vi "Command to Analog Output.vi"() -> ()   [LabVIEW 2019, in "Part of Main VIs.lvlib" / "Command Library.lvlib"]
uses:
  <vilib>/DAQmx/write.llb/DAQmx Write (Analog DBL 1Chan 1Samp).vi
  <extravilib>/ChannelInstances/Tag-bool/Write With Abort.vi
  <extravilib>/ChannelInstances/Tag-str/Write With Abort.vi
  <extravilib>/ChannelInstances/Tag-bool/Read With Abort.vi
  <extravilib>/ChannelInstances/Tag-str/Read With Abort.vi
  <extravilib>/ChannelInstances/Tag-dbl/Write With Abort.vi
  <extravilib>/ChannelInstances/Tag-dbl/Read With Abort.vi
  <extravilib>/ChannelInstances/Tag-str/Instantiate.vi
  <extravilib>/ChannelInstances/Tag-dbl/Instantiate.vi
  <extravilib>/ChannelInstances/Tag-bool/Instantiate.vi
  <extravilib>/ChannelInstances/Tag-bool/EndpointRead.vi
  <extravilib>/ChannelInstances/Tag-str/EndpointRead.vi
  <extravilib>/ChannelInstances/Tag-dbl/Endpoint.vi
  <extravilib>/ChannelInstances/Tag-str/Endpoint.vi
  <vilib>/DAQmx/create/channels.llb/DAQmx Create Channel (AO-Voltage-Basic).vi
  <extravilib>/ChannelInstances/Tag-dbl/EndpointRead.vi
  <vilib>/DAQmx/miscellaneous.llb/DAQmx Fill In Error Info.vi
  <extravilib>/ChannelInstances/Tag-bool/Endpoint.vi
  Command Library.lvlib
  <extravilib>/ChannelInstances/Tag-bool.lvlib
  <resource>/objmgr/daqmx.rc
  <extravilib>/ChannelInstances/Tag-dbl.lvlib
  <extravilib>/ChannelInstances/Tag-str.lvlib
panel:
  out "Numeric 2":dbl
  in  "Numeric":dbl
  out "Waveform Chart":waveform(dbl)(graph)
  in  "stop":bool
  in  "String":string
  out "InterfaceName":string
  out "Voltage Value":dbl format="%e"
  out "BoardName":string
  out "ChannelNo":string
  out "Status":string
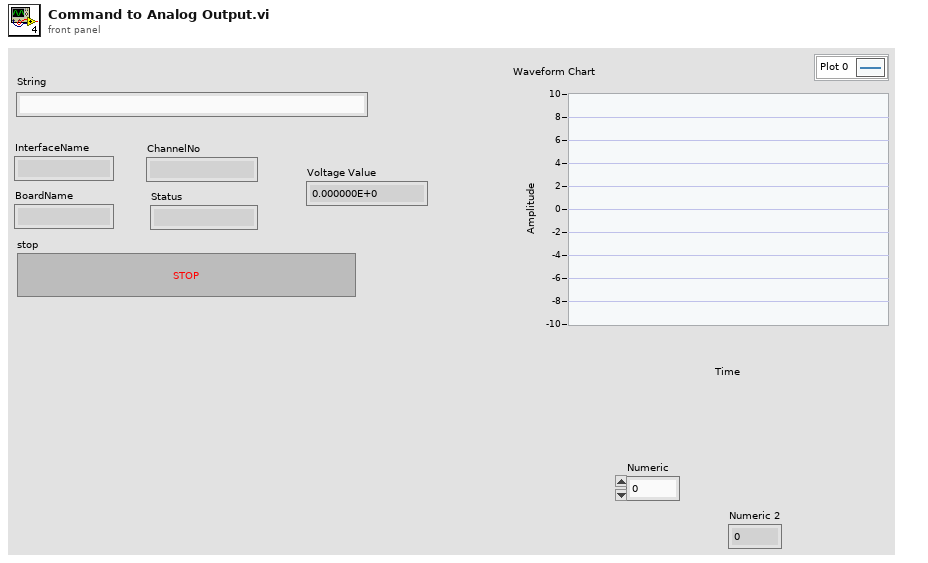
[diagram p1: front panel]
types:
  T1 = typedef "Tag-str.lvlib/))Channel.ctl" = refnum<queue>
  T2 = typedef "Tag-bool.lvlib/))Channel.ctl" = refnum<queue>
  T3 = typedef "Tag-dbl.lvlib/))Channel.ctl" = refnum<queue>
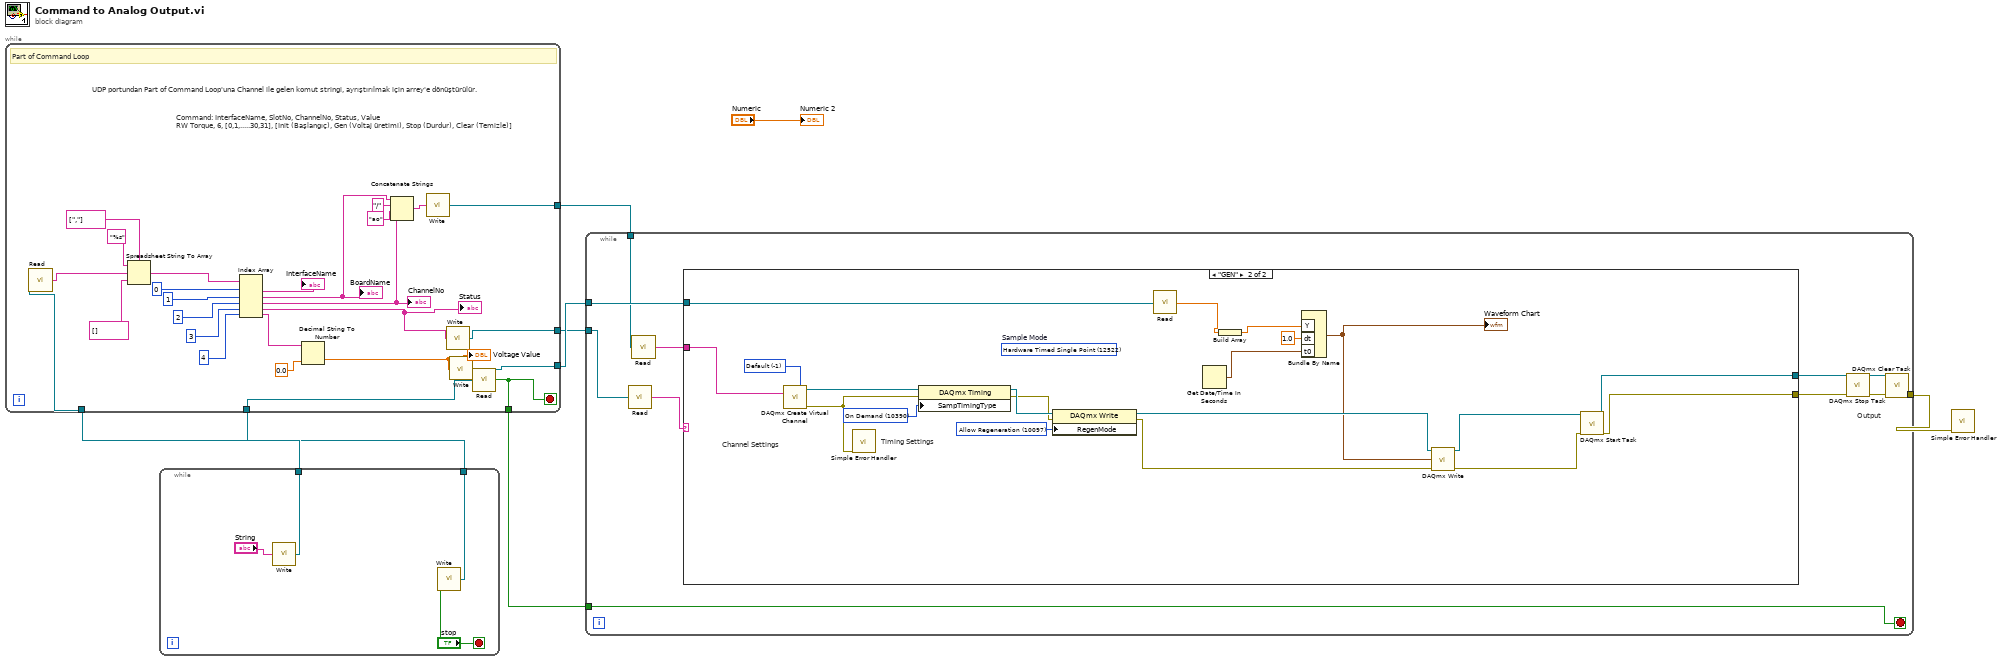
[diagram p0: block diagram]
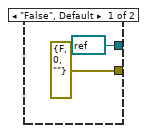
[diagram p2: hidden frame]
diagram:
  n1 = while {
    tunnel: [w11] -> w8
    tunnel: [w9] -> w7
    stop <- "stop" stop-if-true
    n2 = call <extravilib>:"Write.vi"("element"="String") -> ("channel"=w11:T1)  [unwired: 1 out]
    n3 = call <extravilib>:"Write.vi"("element"="stop") -> ("channel"=w9:T2)  [unwired: 1 out]
  }
  n4 = while {
    tunnel: w8 -> [w35]
    tunnel: w7 -> [w26]
    tunnel: [w23] -> w4
    tunnel: [w27] -> w5
    tunnel: [w25] -> w2
    tunnel: [w19] -> w3
    stop <- w25 stop-if-true
    # "UDP portundan Part of Command Loop'una Channel ile gelen komut stringi, ayrıştırılmak için arrey'e dönüştürülür."
    # "Command: InterfaceName, SlotNo, ChannelNo, Status, Value\nRW Torque, 6, [0,1,.....30,31], [Init (Başlangıç), Gen (Voltaj üretimi), Stop (Durdur), Clear (Temizle)]"
    # "Part of Command Loop"
    n5 = call <extravilib>:"Read.vi"("channel"=w35) -> ("element"=w34:string)  [unwired: 1 in, 1 out]
    n6 = Spreadsheet String To Array(delimiter (Tab)=string[] [","], format string="%s", spreadsheet string=w34, array type (2D Dbl)=string[] [] ("Array")) -> (array=w37:string[])
    n7 = Index Array "Index Array"(array=w37, index #1=0 ("index"), index #2=1 ("index"), index #3=2 ("index"), index #4=3 ("index"), index #5=4 ("index")) -> (element #1=→"InterfaceName":string, element #2=w18:string, element #3=w16:string, element #4=w24:string, element #5=w14:string)
    "BoardName" <- w18
    "ChannelNo" <- w16
    "Status" <- w24
    n8 = Decimal String To Number(string=w14, default (0L)=0.0) -> (number=w13:dbl)  [unwired: 1 in, 1 out]
    "Voltage Value" <- w13
    n9 = Concatenate Strings(w18, "/" ("string"), "ao" ("string"), w16) -> (w20:string)
    n10 = call <extravilib>:"Write.vi"("element"=w20) -> ("channel"=w19:T1)  [unwired: 1 out]
    n11 = call <extravilib>:"Write.vi"("element"=w24) -> ("channel"=w23:T1)  [unwired: 1 out]
    n12 = call <extravilib>:"Write.vi"("element"=w13) -> ("channel"=w27:T3)  [unwired: 1 out]
    n13 = call <extravilib>:"Read.vi"("channel"=w26) -> ("element"=w25:bool)  [unwired: 1 in, 1 out]
  }
  n14 = while {
    tunnel: w4 -> [w43]
    tunnel: [w49] -> w6
    tunnel: w5 -> [w44]
    tunnel: w3 -> [w41]
    tunnel: w2 -> [w39]
    stop <- w39 stop-if-true
    # "Output"
    n15 = call <extravilib>:"Read.vi"("channel"=w43) -> ("element"=w42:string)  [unwired: 1 in, 1 out]
    n16 = call <extravilib>:"Read.vi"("channel"=w41) -> ("element"=w40:string)  [unwired: 1 in, 1 out]
    n17 = case shown="\"GEN\"" w42 {
      tunnel: [refnum<k21> refnum ("task out") w63] -> w46
      tunnel: [errorcluster {"status"=FALSE, "code"=0, "source"=""} ("error out") w64] -> w45
      tunnel: w44 -> [_ w67]
      tunnel: w40 -> [_ w52]
      frame "False", Default {
      }
      frame "GEN" {
        w60 = 10097 items=["Allow Regeneration"=10097, "Do Not Allow Regeneration"=10158] ("RegenMode")
        w70 = 10390 items=["Sample Clock"=10388, "Burst Handshake"=12548, "Handshake"=10389, "Implicit"=10451, "On Demand"=10390, "Change Detection"=12504, "Pipelined Sample Clock"=14668] ("SampTimingType")
        w71 = -1 items=["Default"=-1, "RSE"=10083, "Differential"=10106, "Pseudodifferential"=12529] ("output terminal configuration")
        (unwired) 12522 items=["Finite Samples"=10178, "Continuous Samples"=10123, "Hardware Timed Single Point"=12522]  # Sample Mode
        # "Timing Settings"
        # "Channel Settings"
        n18 = call-poly <vilib>:"DAQmx Create Virtual Channel.vi"("output terminal configuration"=w71, "physical channels"=w52) -> ("task out"=w69:refnum<k21>, "error out"=w68:errorcluster)  [unwired: 12 in]
        n19 = call <vilib>:"Simple Error Handler.vi"("error in (no error)"=w68) -> ()  [unwired: 4 in, 5 out]
        n20 = property class="DAQmx Timing"(reference=w69, error in=w68, "SampTimingType"=w70) -> (reference out=w62:refnum<k21>, error out=w61:errorcluster)
        n21 = property class="DAQmx Write"(reference=w62, error in=w61, "RegenMode"=w60) -> (reference out=w59:refnum<k21>, error out=w58:errorcluster)
        n22 = call <extravilib>:"Read.vi"("channel"=w67) -> ("element"=w56:dbl)  [unwired: 1 in, 1 out]
        n23 = Get Date/Time In Seconds() -> (seconds since 1Jan1904=w53:timestamp)
        n24 = Build Array(w56) -> (w55:dbl[])
        n25 = Bundle By Name("Y"=w55, "dt"=1.0, "t0"=w53) -> (w54:waveform(dbl))  [unwired: 1 in]
        "Waveform Chart" <- w54
        n26 = call-poly <vilib>:"DAQmx Write.vi"("task/channels in"=w59, "data"=w54, "error in"=w58) -> ("task out"=w66:refnum<k21>, "error out"=w65:errorcluster)  [unwired: 10 in, 1 out]
        n27 = call <vilib>:"DAQmx Start Task.vi"("task/channels in"=w66, "error in"=w65) -> ("task out"=w63:refnum<k21>, "error out"=w64:errorcluster)  [unwired: 12 in]
      }
    }
    n28 = call <vilib>:"DAQmx Stop Task.vi"("task/channels in"=w46, "error in"=w45) -> ("task out"=w47:refnum<k21>, "error out"=w48:errorcluster)  [unwired: 12 in]
    n29 = call <vilib>:"DAQmx Clear Task.vi"("task in"=w47, "error in"=w48) -> ("error out"=w49:errorcluster)  [unwired: 13 in]
  }
  n30 = call <vilib>:"Simple Error Handler.vi"("error in (no error)"=w6) -> ()  [unwired: 4 in, 5 out]
  "Numeric 2" <- "Numeric"
